vi "Concatenate_Blocks.vi"() -> (5 "Plug in titles":string[](array[string]), 7 "Plug in values":string[](array[string]))   [LabVIEW 2017]
uses:
  <vilib>/Analysis/2dsp.llb/Integral Method.ctl
  Controls/Post_Process.ctl
  Controls/Graph_Type.ctl
  <vilib>/Analysis/baseanly.llb/Mean (DBL).vi
  <vilib>/Analysis/8numeric.llb/1D Numeric Integration.vi
  Globals/Meas_global.vi
  <vilib>/Analysis/NI_AALBase.lvlib
  <vilib>/Analysis/NI_AALPro.lvlib
panel:
  out "Av Sampling Rate":dbl format="%0.2f"
  in  "Calculate Spectra and Histogram?":bool
  out "Integral (u^2)":dbl format="%0.4f"
  in  "integration method":T1 items=["Trapezoidal Rule", "Simpson's Rule", "Simpson's 3/8 Rule", "Bode Rule"]
  in  "PDF":bool=TRUE
  out "nSpectral Averages":i32
  out "Autocorrelation":cluster{dbl, dbl, dbl[]}[](graph)
  in  "No of averged samples in spectra":i32=4096
  out "Spectra":cluster{dbl, dbl, dbl[]}[](graph)
  out "Histogram/Pdf":T2(graph)
  in  "Show Smooth":bool=TRUE
  in  "Save Plots":bool
  in  "Averaging samples":i32=5 min=1 max=1000
  out "Waveform Graph":dbl[][](graph)
  in  "Channels to Plot":i32[](array[ring])=[0] items=["RV (V1)", "RV (V2)", "RV (Inert)", "RV (Reactive)", "RV (V5)", "RV (Sync)", "RV (C)", "Save Nothing"]
  # "Run this VI to update the channel names"
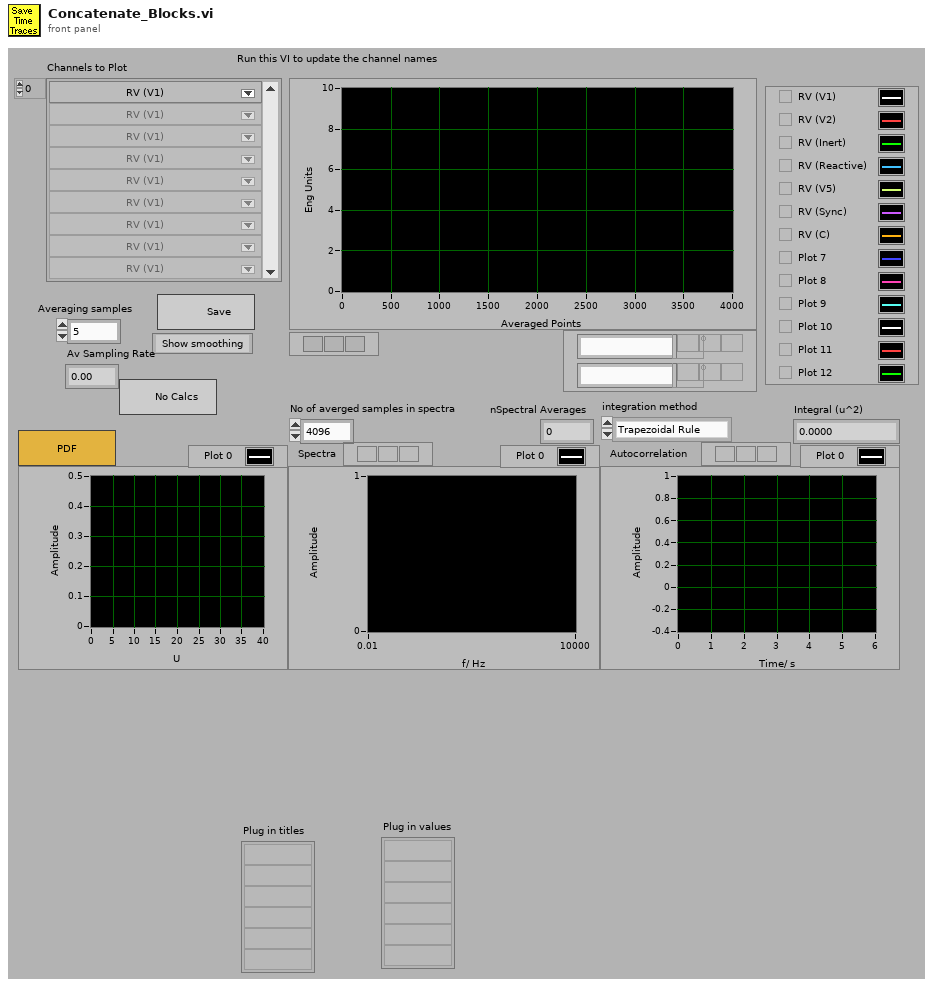
[diagram p1: front panel]
types:
  T1 = typedef "NI_AALPro.lvlib/Integral Method.ctl" = i32
  T2 = cluster{"element":dbl, dbl, "1D histogram or PDF":dbl[]}[]
  T3 = typedef "Analysis_info_cluster.ctl" = cluster{"Colour":u32, "Inst type":T4, "Inst name":string, "Symbol":string, "Code name":string, "Extra Info":string, "Inst Array":T5, "Extra Titles":string[], "Extra Values":string[], "U":dbl, "u^2":dbl, "u^3":dbl, "u^4":dbl, "Skew_u":dbl, "Kurt_u":dbl, "Sd Error in Mean":dbl, "% u'/U":dbl, "X":dbl, "Y":dbl, "Z":dbl, "Timescale integral Estimate":dbl, "Sd Error in Variance":dbl, "Calib File":path, "Calib Constants":dbl[], "Output Position":bool, "Full Stats":bool, "Av Sampling Rate":dbl, "Av No of Samples":dbl, "Total Meas Time (s)":dbl, "ADAM Ch Name":string, "Max value":dbl, "Min value":dbl, "Req Sample Rate Hz":dbl, "Sync Delay Time (s)":dbl, "Ch No":i16, "Device ID":string, "Use Latest Calib":bool, "Port":string}
  T4 = typedef "Inst_type.ctl" = enum16{"Propeller anemometer", "Raw voltage", "Pressure Transducer", "Pitot-static tube", "Preston tube", "Hot wire", "Cross wire 1", "Cross wire 2", "Generic Linear", "Generic Polynomial", "Generic BackPoly", "Fast FID", "Thermocouple", "Cold wire", "Pulsed Wire", "LDA Vel", "LDA Tran time", "LDA Arr time", "Microphone"}
  T5 = typedef "Instrument_Array.ctl" = enum16{"PWA", "LDA", "Analogue"}
  T6 = typedef "Time_Trace_Cluster.ctl" = cluster{"Weighting":dbl[], "Time (s)":dbl[], "Voltage":dbl[], "Eng Values":dbl[]}
  T7 = typedef "Post_Process.ctl" = enum16{"Take New Data", "Post Process Raw Data File"}
  T8 = typedef "Graph_Type.ctl" = enum16{"Show no graph", "Voltage trace", "Velocity trace", "Vel histogram", "Spectrum", "f.E(f) v Log f", "Auto-Corr"}
  T9 = cluster{"Plot 1":u16, "Plot 2":u16, "Save graph":u16, "Plot Type":T8}
  T10 = cluster{"element":dbl, dbl, "1D histogram or PDF":dbl[]}
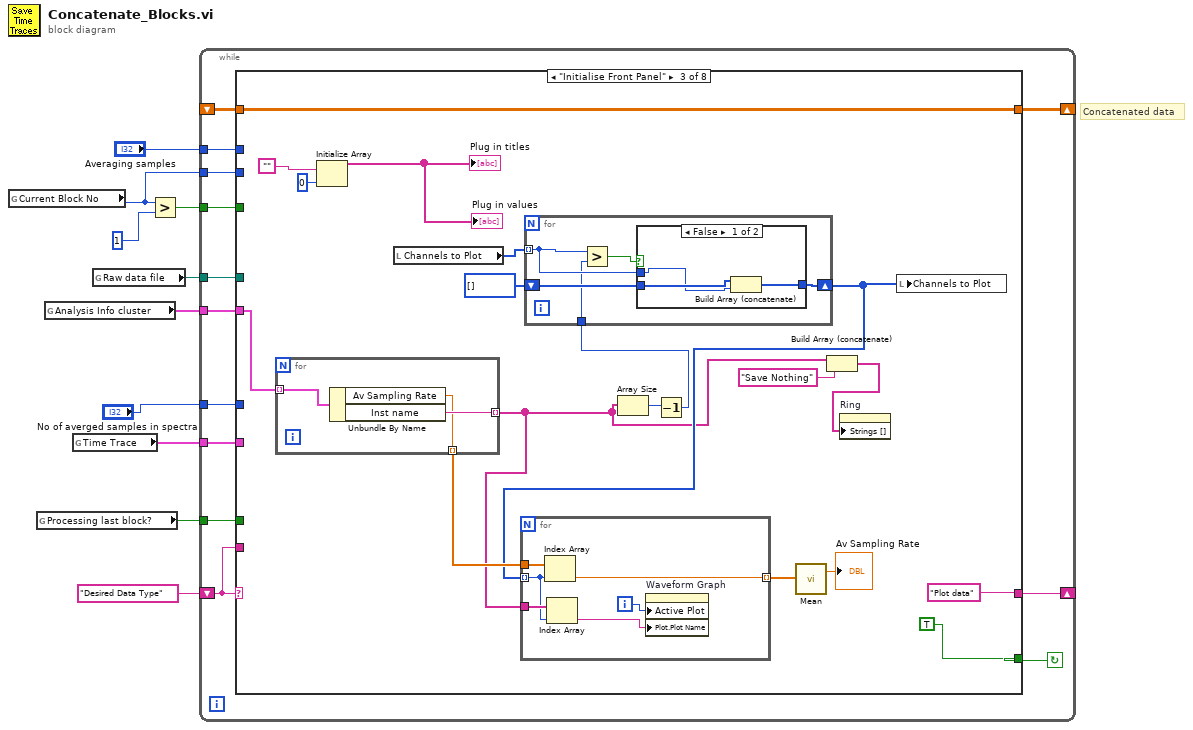
[diagram p0: block diagram]
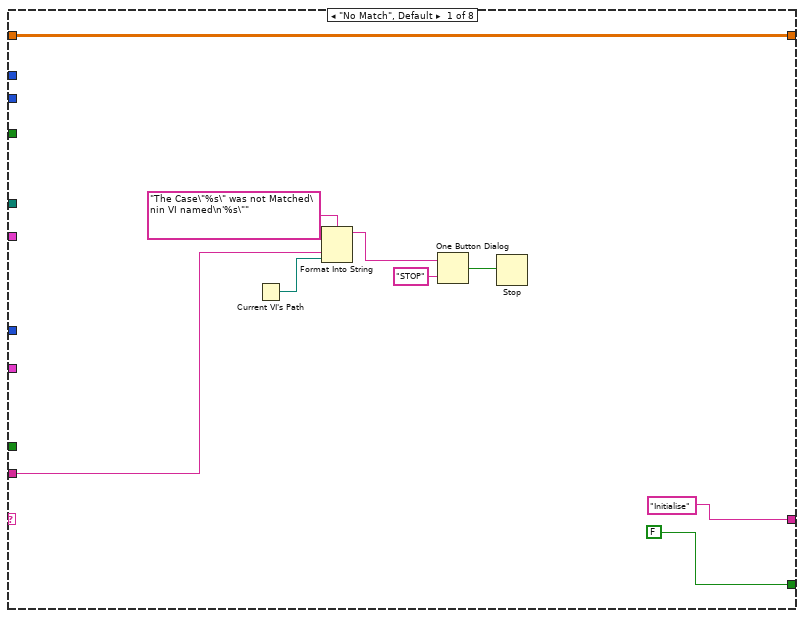
[diagram p2: hidden frame]
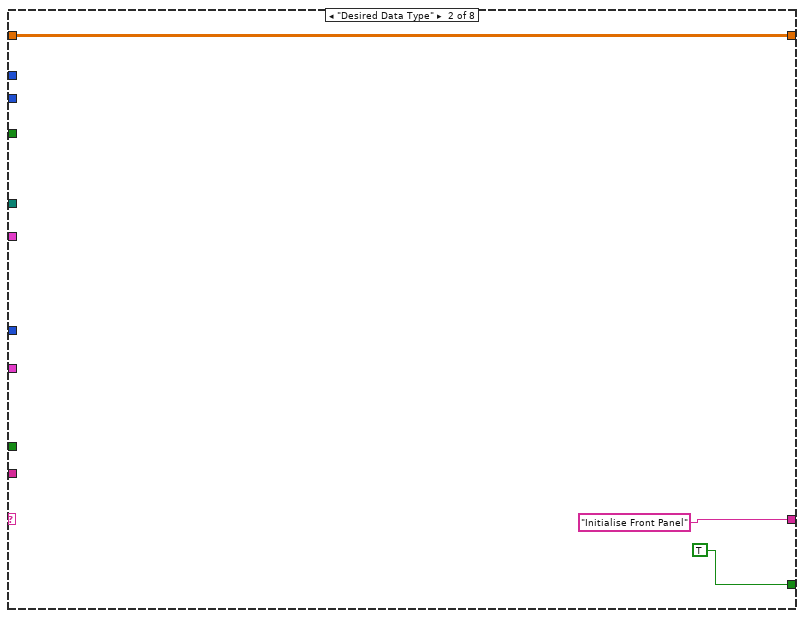
[diagram p3: hidden frame]
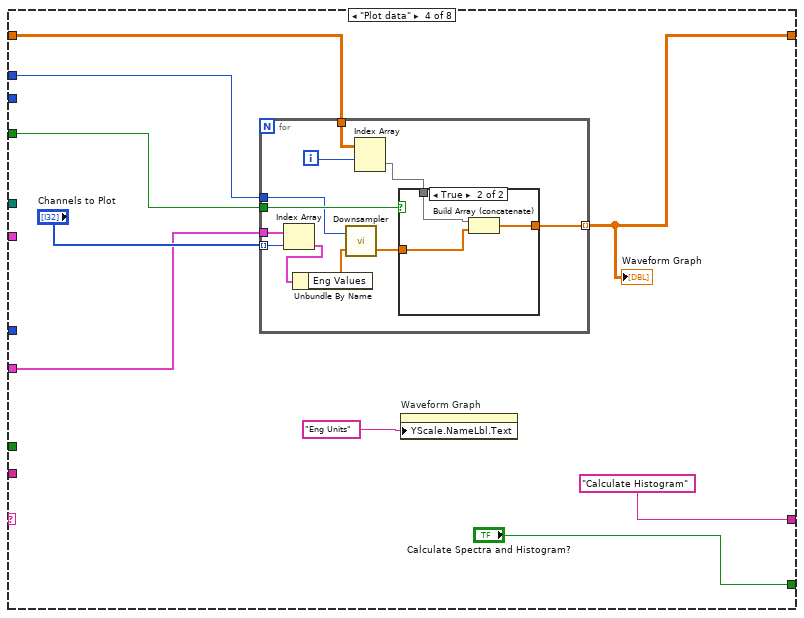
[diagram p5: hidden frame]
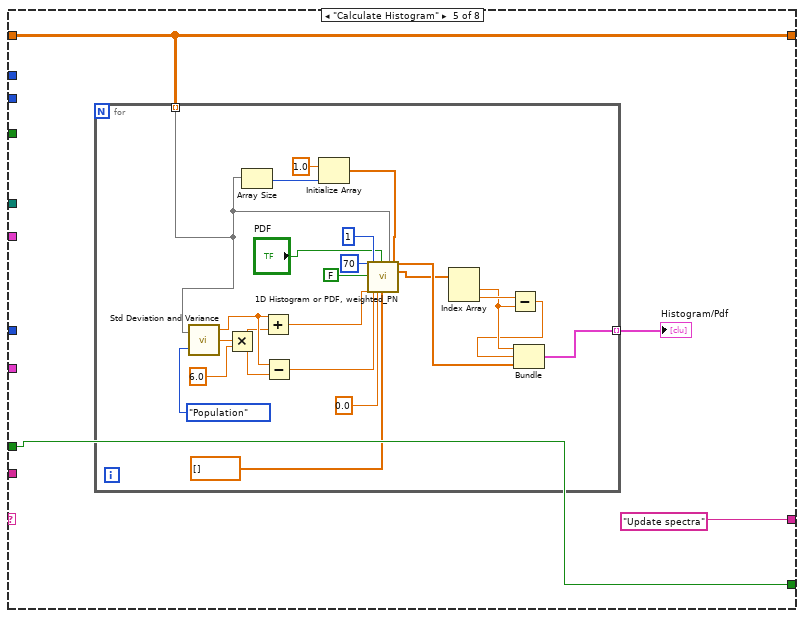
[diagram p7: hidden frame]
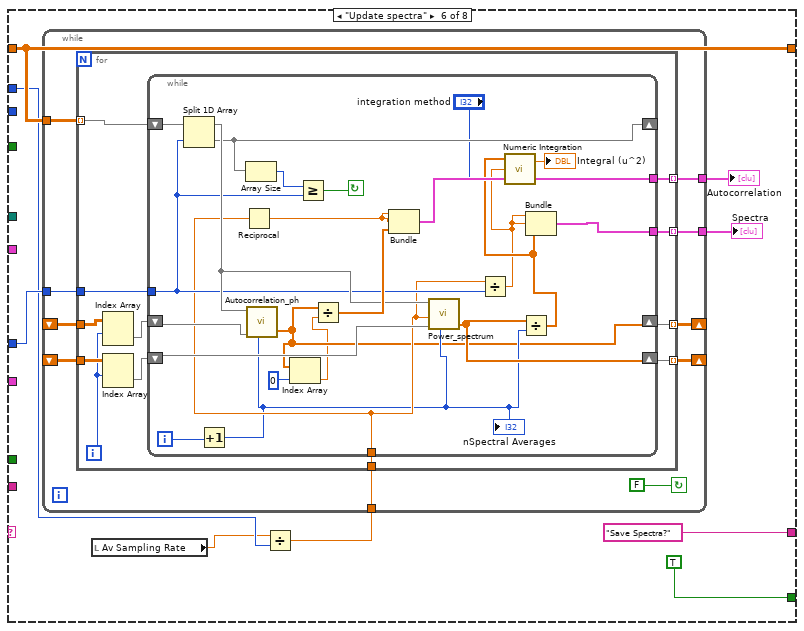
[diagram p8: hidden frame]
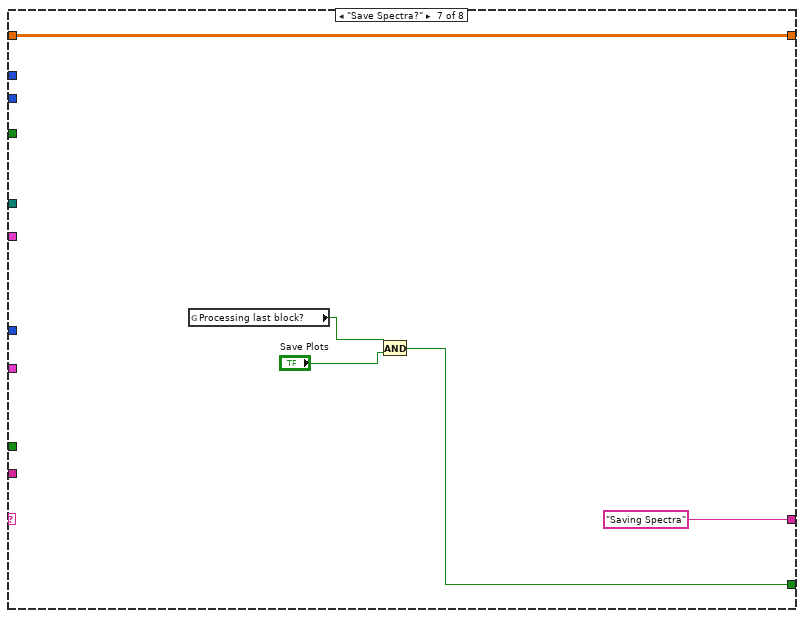
[diagram p9: hidden frame]
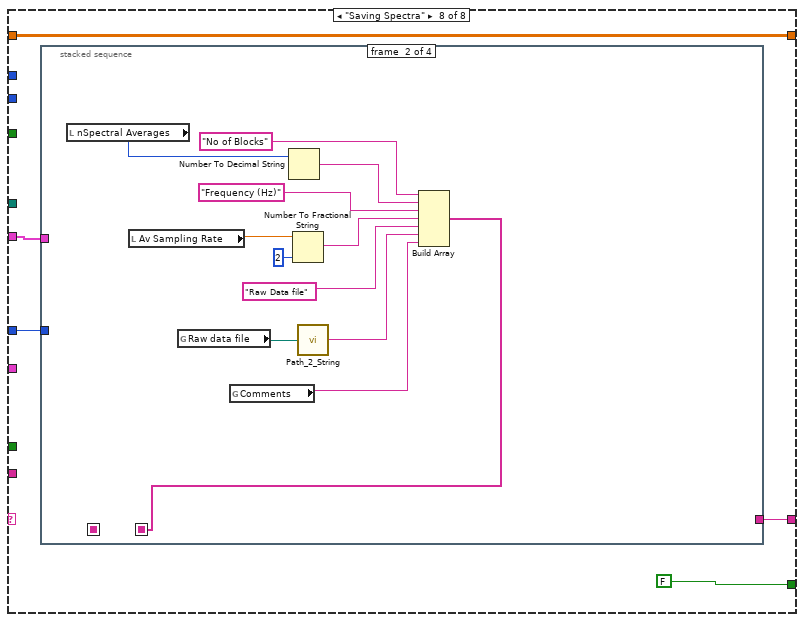
[diagram p10: hidden frame]
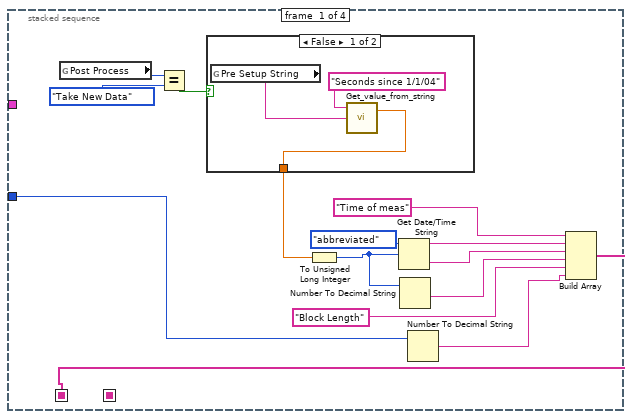
[diagram p11: hidden frame]
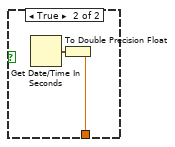
[diagram p12: hidden frame]
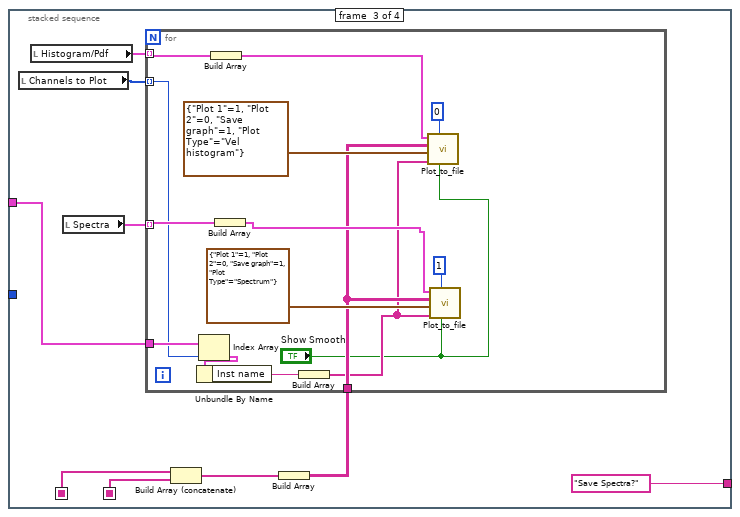
[diagram p13: hidden frame]
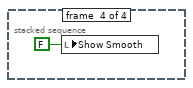
[diagram p14: hidden frame]
diagram:
  # "Concatenated data"
  n1 = global read "Meas_global.vi" "Current Block No"() -> (w7:i32)
  n2 = global read "Meas_global.vi" "Processing last block?"() -> (w1:bool)
  n3 = global read "Meas_global.vi" "Analysis Info cluster"() -> (w6:T3[])
  n4 = global read "Meas_global.vi" "Time Trace"() -> (w3:T6[])
  n5 = global read "Meas_global.vi" "Raw data file"() -> (w9:path)
  n6 = Greater?(x=w7, y=1) -> (0:w5:bool)
  n7 = while {
    shift-left: "Desired Data Type" -> [w21]
    shift-right: [w22] -> _
    tunnel: w9 -> [w20]
    tunnel: w5 -> [w19]
    tunnel: w7 -> [w18]
    tunnel: w6 -> [w17]
    shift-right: [w15] -> _
    shift-left: _ -> [w16]
    tunnel: "No of averged samples in spectra" -> [w14]
    tunnel: w3 -> [w13]
    tunnel: "Averaging samples" -> [w12]
    tunnel: w1 -> [w11]
    stop <- w23 continue-if-true
    n8 = case shown="\"Initialise Front Panel\"" w21 {
      tunnel: [FALSE TRUE TRUE "Calculate Spectra and Histogram?" w97 TRUE ("Calculate Spectra and Histogram?") w177 FALSE ("Calculate Spectra and Histogram?")] -> w23
      tunnel: ["Initialise" "Initialise Front Panel" "Plot data" "Calculate Histogram" ("t") "Update spectra" "Save Spectra?" "Saving Spectra" w185] -> w22
      tunnel: w21 -> [w27 _ _ _ _ _ _ _]
      tunnel: w20 -> [_ _ _ _ _ _ _ _]
      tunnel: w19 -> [_ _ _ w79 _ _ _ _]
      tunnel: w18 -> [_ _ _ _ _ _ _ _]
      tunnel: w17 -> [_ _ w41 _ _ _ _ w184]
      tunnel: w16 -> [w24 w33 w44 w80 w99 w128 w181 w186]
      tunnel: [w24 w33 w44 w77 w99 w128 w181 w186] -> w15
      tunnel: w14 -> [_ _ _ _ _ w129 _ w182]
      tunnel: w13 -> [_ _ _ w73 _ _ _ _]
      tunnel: w12 -> [_ _ _ w72 _ w127 _ _]
      tunnel: w11 -> [_ _ _ _ w97 _ _ _]
      frame "No Match", Default {
        n9 = Current VI's Path() -> (path=w26:path)
        n10 = Format Into String(format string="The Case\"%s\" was not Matched\nin VI named\n'%s\"" ("Format String"), w27, w26) -> (resulting string=w30:string)  [unwired: 2 in, 1 out]
        n11 = One Button Dialog(message=w30, button name ("OK")="STOP") -> (true=w28:bool)
        n12 = Stop(stop? (T)=w28) -> ()
      }
      frame "Desired Data Type" {
      }
      frame "Initialise Front Panel" {
        n13 = for {
          tunnel: w41 -> [w62] mode=indexing
          tunnel: [w61] -> w36 mode=indexing
          tunnel: [w60] -> w40 mode=indexing
          n14 = Unbundle By Name(w62) -> ("Av Sampling Rate"=w60:dbl, "Inst name"=w61:string)
        }
        n15 = Initialize Array("", 0) -> (→"Plug in values" →"Plug in titles":string[])
        n16 = local read "Channels to Plot"() -> (w50:i32[])
        n17 = Array Size(array=w36) -> (size(s)=w46:i32)
        n18 = Decrement(x=w46) -> (x-1=w45:i32)
        n19 = for {
          tunnel: w50 -> [w64] mode=indexing
          shift-right: [w65] -> w39
          shift-left: i32[] [] -> [w66]
          tunnel: w45 -> [w63]
          n20 = Greater?(x=w64, y=w63) -> (0:w67:bool)
          n21 = case shown="False" w67 {
            tunnel: w66 -> [w70 w71]
            tunnel: [w69 w71] -> w65
            tunnel: w64 -> [w68 _]
            frame False {
              n22 = Build Array (concatenate)(w70, w68) -> (w69:i32[])
            }
            frame True {
            }
          }
        }
        n23 = for {
          tunnel: w40 -> [w59]
          tunnel: w39 -> [w56] mode=indexing
          tunnel: [w58] -> w38 mode=indexing
          tunnel: w36 -> [w57]
          i -> [w55]
          n24 = Index Array(array=w59, index=w56) -> (element=w58:dbl)
          n25 = Index Array(array=w57, index=w56) -> (element=w54:string)
          n26 = property on="Waveform Graph" class="WFGraph (strict)"("Active Plot"=w55, "Plot.Plot Name"=w54) -> ()  [unwired: 2 in, 2 out]
        }
        n27 = call-poly <vilib>:"Mean.vi"("X"=w38) -> ("mean"=→"Av Sampling Rate":dbl)  [unwired: 1 out]
        n28 = Build Array (concatenate)(w36, "Save Nothing") -> (w47:string[])
        n29 = property on="Ring" class="Ring (strict)"("Strings []"=w47) -> ()  [unwired: 2 in, 2 out]
        n30 = local write "Channels to Plot"(w39) -> ()
      }
      frame "Plot data" {
        n31 = for {
          tunnel: w73 -> [w91]
          tunnel: "Channels to Plot" -> [w90] mode=indexing
          tunnel: w80 -> [w87]
          tunnel: [w88] -> w77 mode=indexing
          tunnel: w79 -> [w89]
          tunnel: w72 -> [w81]
          i -> [w86]
          n32 = Index Array(array=w91, index=w90) -> (element=w83:T6)
          n33 = Unbundle By Name(w83) -> ("Eng Values"=w82:dbl[])
          n34 = call "Downsampler.vi"("Input Array"=w82, "Averaging samples"=w81) -> ("Downsampled Array"=w84:dbl[])  [unwired: 1 out]
          n35 = Index Array(array=w87, index (row)=w86) -> (element=w85:dbl[])  [unwired: 1 in]
          n36 = case shown="True" w89 {
            tunnel: w85 -> [_ w95]
            tunnel: w84 -> [w92 w94]
            tunnel: [w92 w93] -> w88
            frame False {
            }
            frame True {
              n37 = Build Array (concatenate)(w95, w94) -> (w93:dbl[])
            }
          }
        }
        "Waveform Graph" <- w77
        n38 = property on="Waveform Graph" class="WFGraph (strict)"("YScale.NameLbl.Text"="Eng Units") -> ()  [unwired: 2 in, 2 out]
      }
      frame "Calculate Histogram" {
        n39 = for {
          tunnel: w99 -> [w100] mode=indexing
          tunnel: [w101] -> w96 mode=indexing
          n40 = call <vilib>:"Std Deviation and Variance.vi"("X"=w100, "Weighting (Sample)"=enum16{"Sample", "Population"}."Population") -> ("mean"=w115:dbl, "standard deviation"=w114:dbl)  [unwired: 1 out]
          n41 = Multiply(x=w114, y=6.0) -> (x*y=w112:dbl)
          n42 = Array Size(array=w100) -> (size(s)=w119:i32)
          n43 = Add(x=w115, y=w112) -> (x+y=w110:dbl)
          n44 = Subtract(x=w115, y=w112) -> (x-y=w109:dbl)
          n45 = Initialize Array(1.0 ("element"), w119) -> (w117:dbl[])
          n46 = call "1D Histogram or PDF, weighted_PN.vi"("Nbins"=70, "Mean shift"=FALSE, "max"=w110, "Current block no."=1, "min"=w109, "Shift SumW in"=0.0, "PDF"="PDF", "Shift PDF in"=dbl[] [], "1D data"=w100, "Weights"=w117) -> ("1D histogram or PDF"=w116:dbl[], "bin centre vals."=w105:dbl[])  [unwired: 13 in, 3 out]
          n47 = Index Array(array=w105) -> (element #1=w103:dbl, element #2=w104:dbl)  [unwired: 2 in]
          n48 = Subtract(x=w104, y=w103) -> (x-y=w102:dbl)
          n49 = Bundle("element"=w103, w102, "1D histogram or PDF"=w116) -> (w101:T10)  [unwired: 1 out]
        }
        "Histogram/Pdf" <- w96
      }
      frame "Update spectra" {
        n50 = local read "Av Sampling Rate"() -> (w123:dbl)
        n51 = Divide(x=w123, y=w127) -> (x/y=w126:dbl)
        n52 = while {
          shift-left: _ -> [w138]
          shift-right: [w141] -> _
          tunnel: w129 -> [w139]
          shift-right: [w136] -> _
          shift-left: _ -> [w137]
          tunnel: w128 -> [w135]
          tunnel: w126 -> [w134]
          tunnel: [w133] -> w125
          tunnel: [w132] -> w124
          stop <- FALSE continue-if-true
          n53 = for {
            tunnel: [w150] -> w141 mode=indexing
            tunnel: w139 -> [w153]
            tunnel: w138 -> [w146]
            tunnel: w137 -> [w148]
            tunnel: [w151] -> w136 mode=indexing
            tunnel: w135 -> [w152] mode=indexing
            tunnel: w134 -> [w149]
            tunnel: [w143] -> w133 mode=indexing
            tunnel: [w142] -> w132 mode=indexing
            i -> [w144]
            n54 = Index Array(array=w148, index (row)=w144) -> (element=w147:dbl[])  [unwired: 1 in]
            n55 = Index Array(array=w146, index (row)=w144) -> (element=w145:dbl[])  [unwired: 1 in]
            n56 = while {
              tunnel: w153 -> [w169]
              shift-right: [w163] -> _
              shift-left: w152 -> [w166]
              shift-right: [w174] -> w150
              shift-left: w145 -> [w172]
              shift-right: [w159] -> w151
              shift-left: w147 -> [w173]
              tunnel: w149 -> [w167]
              tunnel: [w165] -> w143
              tunnel: [w164] -> w142
              i -> [w162]
              stop <- w168 continue-if-true
              n57 = Split 1D Array(array=w166, index=w169) -> (first subarray=w171:dbl[], second subarray=w163:dbl[])
              n58 = Increment(x=w162) -> (x+1=w161:i32)
              "nSpectral Averages" <- w161
              n59 = Reciprocal(x=w167) -> (1/x=w176:dbl)
              n60 = Array Size(array=w163) -> (size(s)=w170:i32)
              n61 = call "Autocorrelation_ph.vi"("X"=w171, "Autocorrelation of X"=w173, "Block No"=w161) -> ("Autocorrelation of X"=w159:dbl[])  [unwired: 3 in]
              n62 = Index Array(array=w159, index=0 ("Index")) -> (element=w158:dbl)
              n63 = Greater Or Equal?(x=w170, y=w169) -> (x >= y?=w168:bool)
              n64 = Divide(x=w159, y=w158) -> (x/y=w175:dbl[])
              n65 = Bundle(w176, w176, w175) -> (w165:cluster{dbl, dbl, dbl[]})  [unwired: 1 out]
              n66 = call "Power_spectrum.vi"("U"=w171, "Sampling frequency"=w167, "Spectrum input array"=w172, "Block No"=w161) -> ("Spectrum Accumulator array"=w174:dbl[])  [unwired: 1 in, 2 out]
              n67 = Divide(x=w167, y=w169) -> (x/y=w154:dbl)
              n68 = Divide(x=w174, y=w161) -> (x/y=w155:dbl[])
              n69 = call-poly <vilib>:"Numeric Integration.vi"("integration method"="integration method", "dt"=w154, "Input Array"=w155) -> ("result"=→"Integral (u^2)":dbl)  [unwired: 1 out]
              n70 = Bundle(w154, w154, w155) -> (w164:cluster{dbl, dbl, dbl[]})  [unwired: 1 out]
            }
          }
        }
        "Spectra" <- w124
        "Autocorrelation" <- w125
      }
      frame "Save Spectra?" {
        n71 = global read "Meas_global.vi" "Processing last block?"() -> (w178:bool)
        n72 = And(x=w178, y="Save Plots") -> (x .and. y?=w177:bool)
      }
      frame "Saving Spectra" {
        n73 = stacked-sequence {
          seq-local: [w190 _ _ _] -> [_ _ w225 _]
          seq-local: [_ w210 _ _] -> [_ _ w224 _]
          tunnel: [_ _ "Save Spectra?" _] -> w185
          tunnel: w184 -> [_ _ w219 _]
          tunnel: w182 -> [w188 _ _ _]
          frame #0 {
            n74 = global read "Meas_global.vi" "Post Process"() -> (w192:T7)
            n75 = Equal?(x=w192, y=Post_Process."Take New Data" ("Post Process")) -> (x = y?=w193:bool)
            n76 = case shown="False" w193 {
              tunnel: [w201 w205] -> w194
              frame False {
                n77 = global read "Meas_global.vi" "Pre Setup String"() -> (w202:string)
                n78 = call "Get_value_from_string.vi"("Input string"=w202, "Variable name"="Seconds since 1/1/04") -> ("Value"=w201:dbl)  [unwired: 1 in, 1 out]
              }
              frame True {
                n79 = Get Date/Time In Seconds() -> (seconds since 1Jan1904=w204:timestamp)
                n80 = To Double Precision Float(number=w204) -> (double precision float=w205:dbl)
              }
            }
            n81 = To Unsigned Long Integer(number=w194) -> (unsigned 32bit integer=w198:u32)
            n82 = Get Date/Time String(date format (0)=enum16{"short", "long", "abbreviated"}."abbreviated", seconds (now)=w198) -> (date string=w196:string, time string=w197:string)  [unwired: 1 out]
            n83 = Number To Decimal String(number=w198) -> (decimal integer string=w199:string)  [unwired: 1 out]
            n84 = Number To Decimal String(number=w188) -> (decimal integer string=w187:string)  [unwired: 1 out]
            n85 = Build Array("Time of meas", w196, w197, w199, "Block Length" ("element"), w187) -> (w190:string[])
          }
          frame #1 {
            n86 = local read "nSpectral Averages"() -> (w207:i32)
            n87 = local read "Av Sampling Rate"() -> (w206:dbl)
            n88 = global read "Meas_global.vi" "Raw data file"() -> (w216:path)
            n89 = global read "Meas_global.vi" "Comments"() -> (w215:string)
            n90 = Number To Decimal String(number=w207) -> (decimal integer string=w208:string)  [unwired: 1 out]
            n91 = Number To Fractional String(number=w206, precision (6)=i16 2) -> (F-format string=w213:string)  [unwired: 2 out]
            n92 = call "Path_2_String.vi"("Real Path"=w216) -> ("Path String"=w217:string)
            n93 = Build Array("No of Blocks", w208, "Frequency (Hz)", w213, "Raw Data file", w217, w215) -> (w210:string[])
          }
          frame #2 {
            n94 = local read "Channels to Plot"() -> (w218:i32[])
            n95 = local read "Histogram/Pdf"() -> (w220:T2)
            n96 = local read "Spectra"() -> (w221:cluster{dbl, dbl, dbl[]}[])
            n97 = Build Array (concatenate)(w225, w224) -> (w223:string[])
            n98 = Build Array(w223) -> (w222:string[][])
            n99 = for {
              tunnel: w222 -> [w230]
              tunnel: w221 -> [w236] mode=indexing
              tunnel: w220 -> [w238] mode=indexing
              tunnel: w219 -> [w234]
              tunnel: w218 -> [w233] mode=indexing
              n100 = Index Array(array=w234, index=w233) -> (element=w231:T3)
              n101 = Unbundle By Name(w231) -> ("Inst name"=w232:string)
              n102 = Build Array(w238) -> (w237:T2)
              n103 = Build Array(w236) -> (w235:cluster{dbl, dbl, dbl[]}[])
              n104 = Build Array(w232) -> (w229:string[])
              n105 = call "Plot_to_file.vi"("Show Smooth"="Show Smooth", "Start trace No"=0, "Trace names"=w229, "Graph"=T9 {"Plot 1"=1, "Plot 2"=0, "Save graph"=1, "Plot Type"=enum."Vel histogram"}, "Plot file label"=w230, "Plot data"=w237) -> ()  [unwired: 6 out]
              n106 = call "Plot_to_file.vi"("Show Smooth"="Show Smooth", "Start trace No"=1, "Trace names"=w229, "Graph"=T9 {"Plot 1"=1, "Plot 2"=0, "Save graph"=1, "Plot Type"=enum."Spectrum"}, "Plot file label"=w230, "Plot data"=w235) -> ()  [unwired: 6 out]
            }
          }
          frame #3 {
            n107 = local write "Show Smooth"(FALSE ("Show Smooth")) -> ()
          }
        }
      }
    }
  }
